vi "Autonomous Independent.vi"() -> ()   [LabVIEW 2016]
doc: "This VI is called when autonomous begins, and will automatically be terminated when autonomous ends. You can carry out timed or sensor driven robot movement independently without needing to return to the caller."
uses:
  <vilib>/Rock Robotics/WPI/Utilities/WPI_GetSetVariantRefNum.vi
  <vilib>/Rock Robotics/Network Tables/NT Write Numeric Array.vi
  Robot Global Data.vi
  <vilib>/Rock Robotics/Network Tables/NT Read String.vi
  <vilib>/Rock Robotics/WPI/RobotDrive/WPI_RobotDriveArcadeDrive_Standard(NoSaturation).vi
panel:
  out "Current Movement, for debugging":T1 {"Y Joystick Value" scale=1.0..-1.0; "X Joystick Value" scale=-1.0..1.0}
  in  "Array of robot movements":T2(array[cluster])=[{"X Joystick Value"=0.39393939393939403, "Y Joystick Value"=0.0, "Delay (sec)"=1.0, "Movement Name"="turn"}, {"X Joystick Value"=-0.3737373737373737, "Y Joystick Value"=0.0, "Delay (sec)"=1.0, "Movement Name"="turn back"}] {"Y Joystick Value" scale=1.0..-1.0; "X Joystick Value" scale=-1.0..1.0}
  # "Be sure to right-click and choose Data Operations>>Make Current Value default if you want to save the array values with the VI"
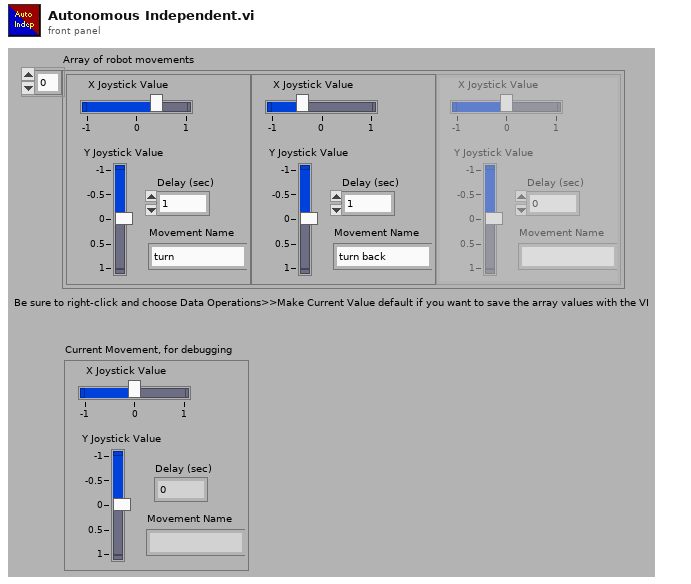
[diagram p1: front panel]
types:
  T1 = cluster{"X Joystick Value":dbl, "Y Joystick Value":dbl, "Delay (sec)":dbl, "Movement Name":string}
  T2 = cluster{"X Joystick Value":dbl, "Y Joystick Value":dbl, "Delay (sec)":dbl, "Movement Name":string}[]
  T3 = cluster{"Current Gear":enum16{"Low", "High"}, "Gear Shift State":enum16{"Low", "Shifting", "High"}}
  T4 = cluster{"Current Position":enum16{"Closed", "Open"}, "Current State":enum16{"Closed", "Shifting", "Open"}}
  T5 = typedef "WPI_RobotDriveDevRef.ctl" = cluster{"DevStatus":errorcluster, "Motors[]":T6[], "Square Inputs":bool, "Max Output":dbl}
  T6 = typedef "WPI_MotorControlDeviceRef.ctl" = cluster{"DeviceStatus":errorcluster, "Type":T7, "PWM":cluster{"PWM Channel":T8, "DeadBand":T9}, "CAN":cluster{"Device Number":u8, "SetOutput VI Ref":variant, "GetOutput VI Ref":variant, "Enable VI Ref":variant, "Disable VI Ref":variant, "Data":variant}, "Invert":bool}
  T7 = typedef "WPI_MotorControlType.ctl" = enum16{"PWM", "CAN"}
  T8 = typedef "FPGA_DIOPWMChannel.ctl" = enum8{"PWM 0", "PWM 1", "PWM 2", "PWM 3", "PWM 4", "PWM 5", "PWM 6", "PWM 7", "PWM 8", "PWM 9", "PWM MXP 0", "PWM MXP 1", "PWM MXP 2", "PWM MXP 3", "PWM MXP 4", "PWM MXP 5", "PWM MXP 6", "PWM MXP 7", "PWM MXP 8", "PWM MXP 9", "Invalid"}
  T9 = typedef "WPI_PWMDeadband.ctl" = cluster{"Name":string, "maxPositivePwm":i32, "minPositivePwm":i32, "centerPwm":i32, "maxNegativePwm":i32, "minNegativePwm":i32, "angularRange":u16}
  T10 = typedef "WPI_JoystickDevRef.ctl" = cluster{"Device":T11}
  T11 = typedef "WPI_JoystickDeviceEnum.ctl" = enum16{"USB 0", "USB 1", "USB 2", "USB 3", "USB 4", "USB 5"}
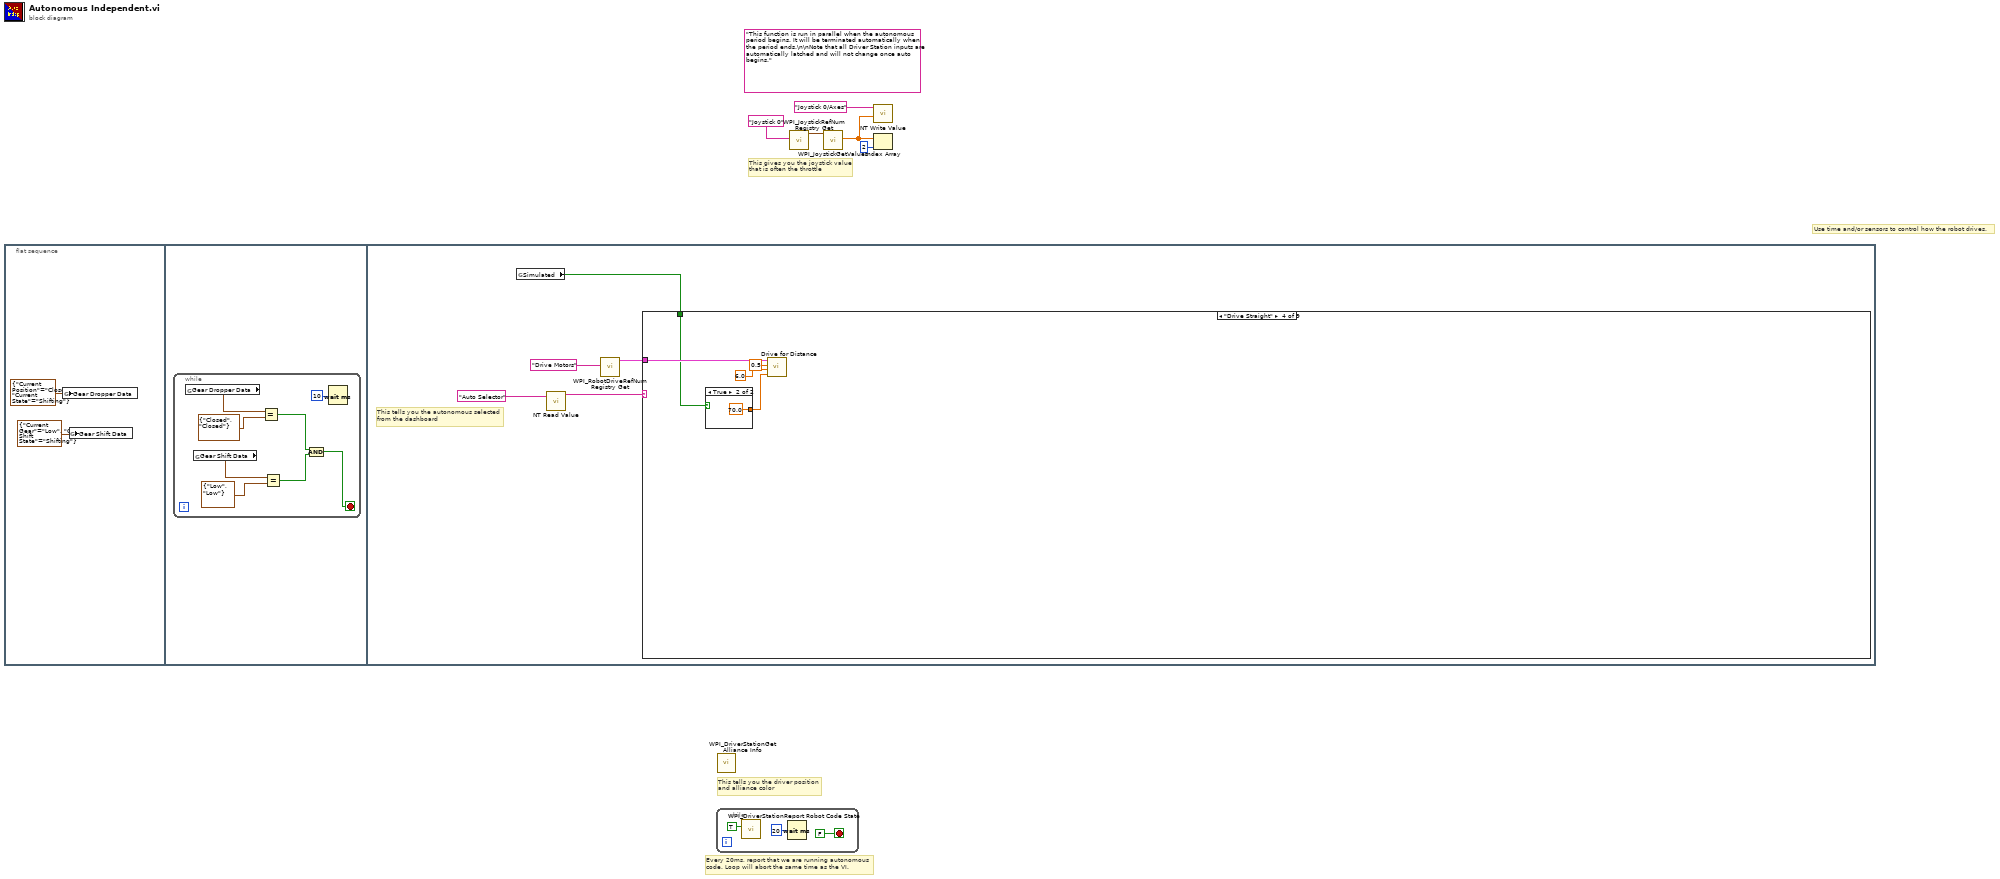
[diagram p0: block diagram]
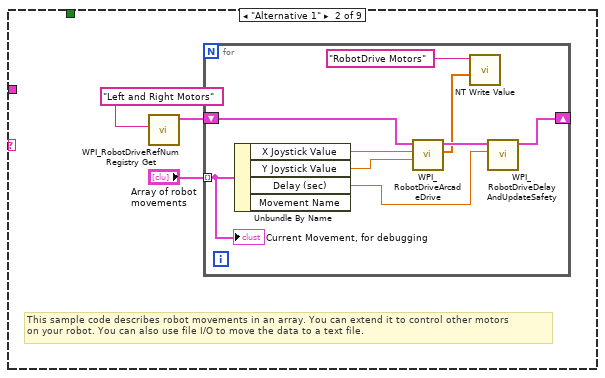
[diagram p3: hidden frame]
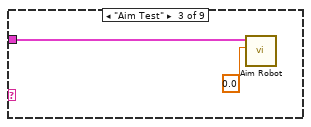
[diagram p4: hidden frame]
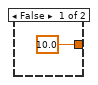
[diagram p5: hidden frame]
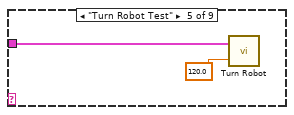
[diagram p6: hidden frame]
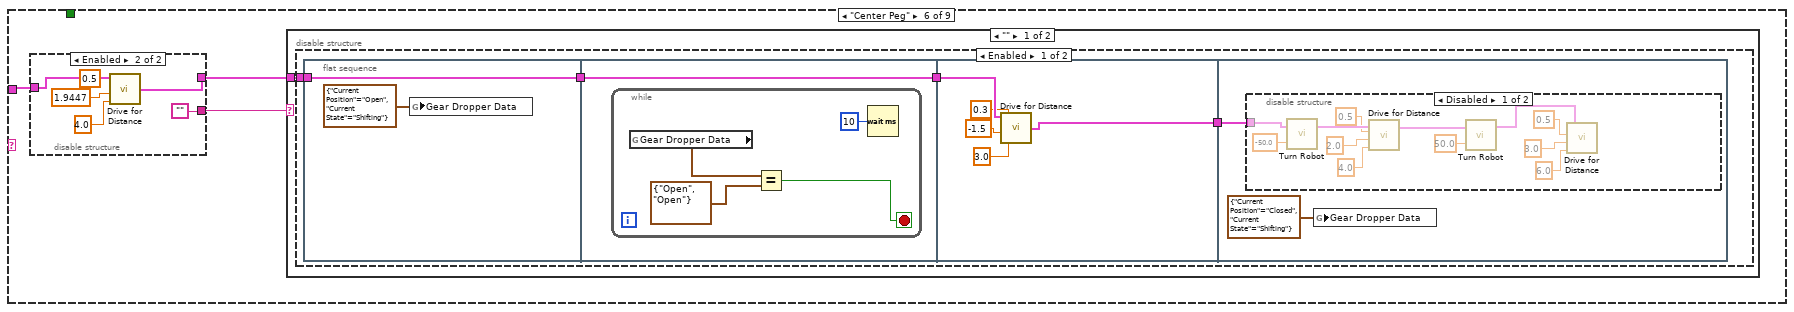
[diagram p7: hidden frame]
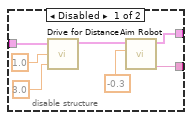
[diagram p8: hidden frame]
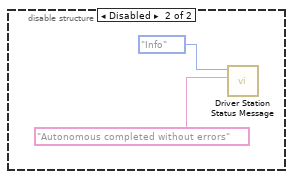
[diagram p10: hidden frame]
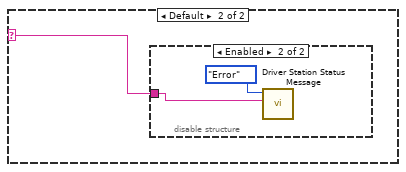
[diagram p11: hidden frame]
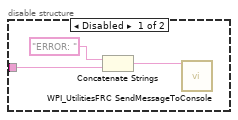
[diagram p12: hidden frame]
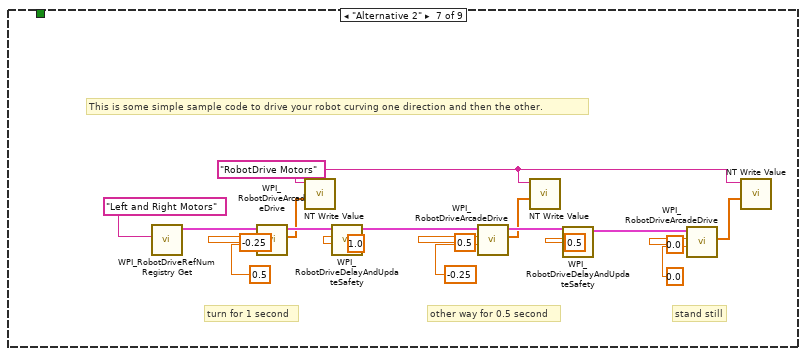
[diagram p13: hidden frame]
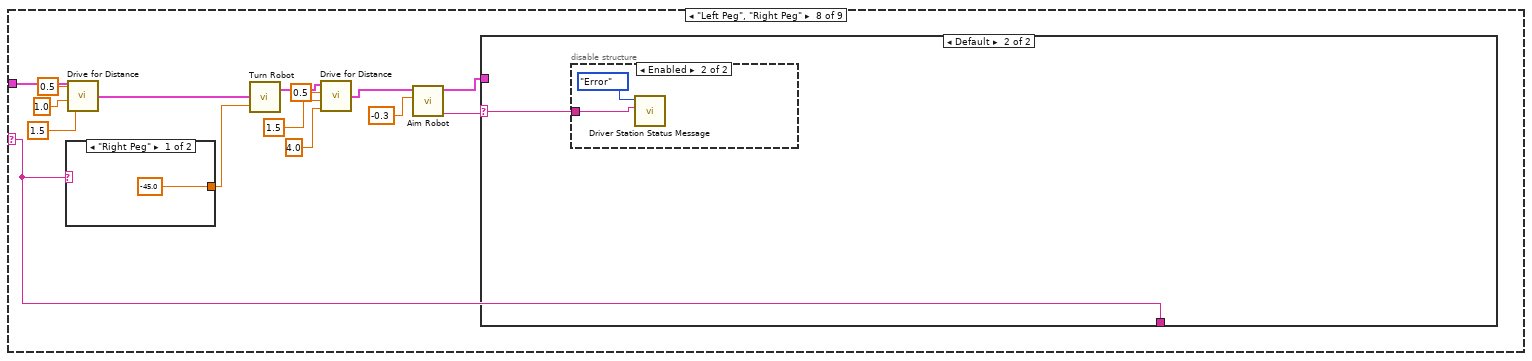
[diagram p14: hidden frame]
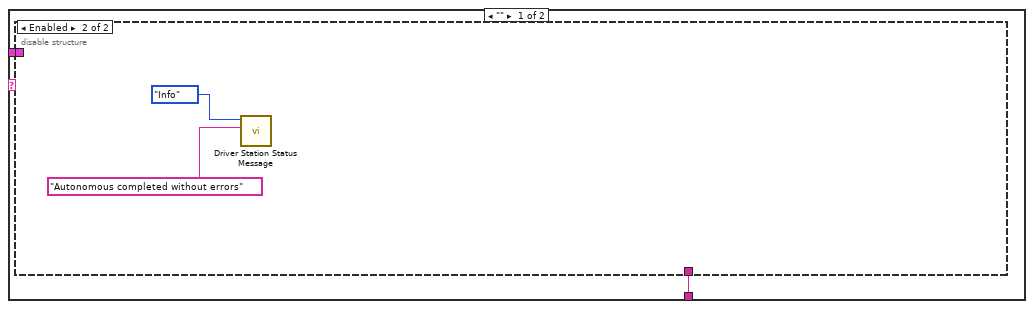
[diagram p15: hidden frame]
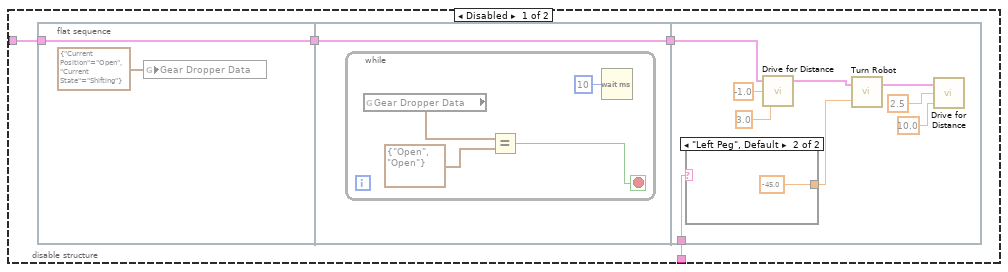
[diagram p16: hidden frame]
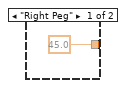
[diagram p17: hidden frame]
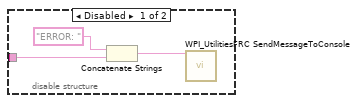
[diagram p18: hidden frame]
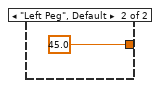
[diagram p19: hidden frame]
diagram:
  (unwired) "This function is run in parallel when the autonomous period begins. It will be terminated automatically when the period ends.\n\nNote that all Driver Station inputs are automatically latched and will not change once auto begins."
  # "Every 20ms, report that we are running autonomous\ncode. Loop will abort the same time as the VI."
  # "This gives you the joystick value\nthat is often the throttle"
  # "Use time and/or sensors to control how the robot drives."
  # "This tells you the driver position\nand alliance color"
  n1 = flat-sequence {
    frame #0 {
      n2 = global write "Robot Global Data.vi" "Gear Dropper Data"(T4 {"Current Position"=enum."Closed", "Current State"=enum."Shifting"} ("Gear Dropper Data")) -> ()
      n3 = global write "Robot Global Data.vi" "Gear Shift Data"(T3 {"Current Gear"=enum."Low", "Gear Shift State"=enum."Shifting"} ("Gear Shift Data")) -> ()
    }
    frame #1 {
      n4 = while {
        stop <- w8 stop-if-true
        n5 = global read "Robot Global Data.vi" "Gear Dropper Data"() -> (w15:T4)
        n6 = global read "Robot Global Data.vi" "Gear Shift Data"() -> (w12:T3)
        n7 = Equal?(x=w15, y=T4 {"Current Position"=enum."Closed", "Current State"=enum."Closed"}) -> (x = y?=w9:bool)
        n8 = Equal?(x=w12, y=T3 {"Current Gear"=enum."Low", "Gear Shift State"=enum."Low"}) -> (x = y?=w10:bool)
        n9 = And(x=w9, y=w10) -> (x .and. y?=w8:bool)
        n10 = Wait (ms)(milliseconds to wait=u32 10) -> ()  [unwired: 1 out]
      }
    }
    frame #2 {
      # "This tells you the autonomous selected\nfrom the dashboard"
      n11 = global read "Robot Global Data.vi" "Simulated"() -> (w16:bool)
      n12 = call-poly <vilib>:"NT Read Value.vi"("Name"="Auto Selector") -> ("String"=w18:string)  [unwired: 9 in, 1 out]
      n13 = call <vilib>:"WPI_RobotDriveRefNum Registry Get.vi"("refnum name"="Drive Motors") -> ("RobotDriveDevRef"=w20:T5)  [unwired: 9 in, 1 out]
      n14 = case shown="\"Drive Straight\"" w18 {
        selector: w18 -> [_ _ _ _ _ _ _ w124 _]
        tunnel: w20 -> [_ _ w33 w39 w43 w46 _ w129 _]
        tunnel: w16 -> [_ _ _ w35 _ _ _ _ _]
        frame Default {
          # "You can put your main auto here, or you can right-click on the case and make any\nother frame be the default case."
          # "This is the frame that will execute if no selection is made, or if it is not recognized"
        }
        frame "Alternative 1" {
          # "This sample code describes robot movements in an array. You can extend it to control other motors\non your robot. You can also use file I/O to move the data to a text file."
          n15 = call <vilib>:"WPI_RobotDriveRefNum Registry Get.vi"("refnum name"="Left and Right Motors") -> ("RobotDriveDevRef"=w22:T5)  [unwired: 1 in, 9 out]
          n16 = for {
            shift-right: [w30] -> _
            shift-left: w22 -> [w31]
            tunnel: "Array of robot movements" -> [w26] mode=indexing
            n17 = Unbundle By Name(w26) -> ("X Joystick Value"=w29:dbl, "Y Joystick Value"=w28:dbl, "Delay (sec)"=w27:dbl)  [unwired: 1 out]
            n18 = call-poly <vilib>:"WPI_RobotDriveArcadeDrive.vi"("Y axis value"=w28, "X axis value"=w29, "RobotDriveDevRef"=w31) -> ("Motor Values"=w24:dbl[], "RobotDriveDevRef"=w32:T5)  [unwired: 1 in, 6 out]
            n19 = call-poly <vilib>:"NT Write Value.vi"("Numeric Array"=w24, "Name"="RobotDrive Motors") -> ()  [unwired: 9 in, 1 out]
            n20 = call <vilib>:"WPI_RobotDriveDelayAndUpdateSafety.vi"("Delay (s)"=w27, "RobotDriveDevRef"=w32) -> ("RobotDriveDevRef 2"=w30:T5)  [unwired: 8 in, 1 out]
            "Current Movement, for debugging" <- w26
          }
        }
        frame "Aim Test" {
          n21 = call "Aim Robot.vi"("Drive Speed"=0.0, "RobotDriveDevRef"=w33) -> ()  [unwired: 8 in, 2 out]
        }
        frame "Drive Straight" {
          n22 = case shown="True" w35 {
            tunnel: [10.0 ("Timeout (s)") 70.0 ("Timeout (s)")] -> w37
            frame False {
            }
            frame True {
            }
          }
          n23 = call "Drive for Distance.vi"("Timeout (s)"=w37, "Distance (m)"=6.0, "Max Speed"=0.5, "RobotDriveDevRef"=w39) -> ()  [unwired: 1 out]
        }
        frame "Turn Robot Test" {
          n24 = call "Turn Robot.vi"("Turn Angle"=120.0, "RobotDriveDevRef"=w43) -> ()  [unwired: 1 in, 1 out]
        }
        frame "Center Peg" {
          n25 = disable-structure shown="Enabled" {
            disable-tunnel: w46 -> [w53 w56]
            disable-tunnel: [w48 w55] -> w45
            disable-tunnel: [w47 ""] -> w44
            frame Disabled {
              n26 = call "Drive for Distance.vi"("Timeout (s)"=3.0, "Distance (m)"=1.0, "RobotDriveDevRef"=w53) -> ("RobotDriveDevRef Out"=w50:T5)  [unwired: 2 in]
              n27 = call "Aim Robot.vi"("Drive Speed"=-0.3, "RobotDriveDevRef"=w50) -> ("Error Out"=w47:string, "RobotDriveDevRef Out"=w48:T5)  [unwired: 8 in]
            }
            frame Enabled {
              n28 = call "Drive for Distance.vi"("Timeout (s)"=4.0, "Distance (m)"=1.9447, "Max Speed"=0.5, "RobotDriveDevRef"=w56) -> ("RobotDriveDevRef Out"=w55:T5)
            }
          }
          n29 = case shown="\"\"" w44 {
            selector: w44 -> [_ w93]
            tunnel: w45 -> [w60 _]
            frame "" {
              n30 = disable-structure shown="Enabled" {
                disable-tunnel: w60 -> [w62 _]
                frame Enabled {
                  n31 = flat-sequence {
                    tunnel: [w65] -> w64
                    tunnel: w62 -> [w65]
                    tunnel: [w67] -> w63
                    tunnel: w64 -> [w67]
                    tunnel: w63 -> [w74]
                    tunnel: [w73] -> w61
                    tunnel: w61 -> [w77]
                    frame #0 {
                      n32 = global write "Robot Global Data.vi" "Gear Dropper Data"(T4 {"Current Position"=enum."Open", "Current State"=enum."Shifting"} ("Gear Dropper Data")) -> ()
                    }
                    frame #1 {
                      n33 = while {
                        stop <- w69 stop-if-true
                        n34 = global read "Robot Global Data.vi" "Gear Dropper Data"() -> (w71:T4)
                        n35 = Equal?(x=w71, y=T4 {"Current Position"=enum."Open", "Current State"=enum."Open"}) -> (x = y?=w69:bool)
                        n36 = Wait (ms)(milliseconds to wait=u32 10) -> ()  [unwired: 1 out]
                      }
                    }
                    frame #2 {
                      n37 = call "Drive for Distance.vi"("Timeout (s)"=3.0, "Distance (m)"=-1.5, "Max Speed"=0.3, "RobotDriveDevRef"=w74) -> ("RobotDriveDevRef Out"=w73:T5)
                    }
                    frame #3 {
                      n38 = disable-structure shown="Disabled" {
                        disable-tunnel: w77 -> [w90 _]
                        frame Disabled {
                          n39 = call "Turn Robot.vi"("Turn Angle"=-50.0, "RobotDriveDevRef"=w90) -> ("RobotDriveDevRef Out"=w88:T5)  [unwired: 1 in]
                          n40 = call "Drive for Distance.vi"("Timeout (s)"=4.0, "Distance (m)"=2.0, "Max Speed"=0.5, "RobotDriveDevRef"=w88) -> ("RobotDriveDevRef Out"=w84:T5)
                          n41 = call "Turn Robot.vi"("Turn Angle"=50.0, "RobotDriveDevRef"=w84) -> ("RobotDriveDevRef Out"=w79:T5)  [unwired: 1 in]
                          n42 = call "Drive for Distance.vi"("Timeout (s)"=6.0, "Distance (m)"=3.0, "Max Speed"=0.5, "RobotDriveDevRef"=w79) -> ()  [unwired: 1 out]
                        }
                        frame Enabled {
                        }
                      }
                      n43 = global write "Robot Global Data.vi" "Gear Dropper Data"(T4 {"Current Position"=enum."Closed", "Current State"=enum."Shifting"} ("Gear Dropper Data")) -> ()
                    }
                  }
                }
                frame Disabled {
                  n44 = call "Driver Station Status Message.vi"("Message"="Autonomous completed without errors", "Message Type"=enum16{"Error", "Warning", "Info"}."Info") -> ()  [unwired: 10 in]
                }
              }
            }
            frame Default {
              n45 = disable-structure shown="Enabled" {
                disable-tunnel: w93 -> [w94 w97]
                frame Disabled {
                  n46 = Concatenate Strings("ERROR: " ("string"), w94) -> (w95:string)
                  n47 = call <vilib>:"WPI_UtilitiesFRC SendMessageToConsole.vi"("Message"=w95) -> ()  [unwired: 14 in, 1 out]
                }
                frame Enabled {
                  n48 = call "Driver Station Status Message.vi"("Message"=w97, "Message Type"=enum16{"Error", "Warning", "Info"}."Error") -> ()  [unwired: 10 in]
                }
              }
            }
          }
        }
        frame "Alternative 2" {
          w100 = "RobotDrive Motors" ("Name")
          # "This is some simple sample code to drive your robot curving one direction and then the other."
          # "stand still"
          # "other way for 0.5 second"
          # "turn for 1 second"
          n49 = call <vilib>:"WPI_RobotDriveRefNum Registry Get.vi"("refnum name"="Left and Right Motors") -> ("RobotDriveDevRef"=w116:T5)  [unwired: 1 in, 9 out]
          n50 = call-poly <vilib>:"WPI_RobotDriveArcadeDrive.vi"("Y axis value"=0.5 ("X axis value"), "X axis value"=-0.25, "RobotDriveDevRef"=w116) -> ("Motor Values"=w99:dbl[], "RobotDriveDevRef"=w109:T5)  [unwired: 1 in, 6 out]
          n51 = call-poly <vilib>:"NT Write Value.vi"("Numeric Array"=w99, "Name"=w100) -> ()  [unwired: 9 in, 1 out]
          n52 = call <vilib>:"WPI_RobotDriveDelayAndUpdateSafety.vi"("Delay (s)"=1.0, "RobotDriveDevRef"=w109) -> ("RobotDriveDevRef 2"=w110:T5)  [unwired: 8 in, 1 out]
          n53 = call-poly <vilib>:"WPI_RobotDriveArcadeDrive.vi"("Y axis value"=-0.25 ("X axis value"), "X axis value"=0.5, "RobotDriveDevRef"=w110) -> ("Motor Values"=w101:dbl[], "RobotDriveDevRef"=w111:T5)  [unwired: 1 in, 6 out]
          n54 = call-poly <vilib>:"NT Write Value.vi"("Numeric Array"=w101, "Name"=w100) -> ()  [unwired: 9 in, 1 out]
          n55 = call <vilib>:"WPI_RobotDriveDelayAndUpdateSafety.vi"("Delay (s)"=0.5, "RobotDriveDevRef"=w111) -> ("RobotDriveDevRef 2"=w112:T5)  [unwired: 8 in, 1 out]
          n56 = call-poly <vilib>:"WPI_RobotDriveArcadeDrive.vi"("Y axis value"=0.0 ("X axis value"), "X axis value"=0.0, "RobotDriveDevRef"=w112) -> ("Motor Values"=w102:dbl[])  [unwired: 1 in, 7 out]
          n57 = call-poly <vilib>:"NT Write Value.vi"("Numeric Array"=w102, "Name"=w100) -> ()  [unwired: 9 in, 1 out]
        }
        frame "Left Peg", "Right Peg" {
          n58 = case shown="\"Right Peg\"" w124 {
            tunnel: [-45.0 45.0] -> w127
            frame "Right Peg" {
            }
            frame "Left Peg", Default {
            }
          }
          n59 = call "Drive for Distance.vi"("Timeout (s)"=1.5, "Distance (m)"=1.0, "Max Speed"=0.5, "RobotDriveDevRef"=w129) -> ("RobotDriveDevRef Out"=w128:T5)
          n60 = call "Turn Robot.vi"("Turn Angle"=w127, "RobotDriveDevRef"=w128) -> ("RobotDriveDevRef Out"=w122:T5)  [unwired: 1 in]
          n61 = call "Drive for Distance.vi"("Timeout (s)"=4.0, "Distance (m)"=1.5, "Max Speed"=0.5, "RobotDriveDevRef"=w122) -> ("RobotDriveDevRef Out"=w121:T5)
          n62 = call "Aim Robot.vi"("Drive Speed"=-0.3, "RobotDriveDevRef"=w121) -> ("Error Out"=w123:string, "RobotDriveDevRef Out"=w125:T5)  [unwired: 8 in]
          n63 = case shown="Default" w123 {
            selector: w123 -> [_ w158]
            tunnel: w125 -> [w133 _]
            tunnel: w124 -> [w132 _]
            frame "" {
              n64 = disable-structure shown="Enabled" {
                disable-tunnel: w133 -> [w135 _]
                disable-tunnel: w132 -> [w134 _]
                frame Disabled {
                  n65 = flat-sequence {
                    tunnel: [w138] -> w137
                    tunnel: w135 -> [w138]
                    tunnel: [w140] -> w136
                    tunnel: w137 -> [w140]
                    tunnel: w136 -> [w147]
                    tunnel: w134 -> [w145]
                    frame #0 {
                      n66 = global write "Robot Global Data.vi" "Gear Dropper Data"(T4 {"Current Position"=enum."Open", "Current State"=enum."Shifting"} ("Gear Dropper Data")) -> ()
                    }
                    frame #1 {
                      n67 = while {
                        stop <- w142 stop-if-true
                        n68 = global read "Robot Global Data.vi" "Gear Dropper Data"() -> (w144:T4)
                        n69 = Equal?(x=w144, y=T4 {"Current Position"=enum."Open", "Current State"=enum."Open"}) -> (x = y?=w142:bool)
                        n70 = Wait (ms)(milliseconds to wait=u32 10) -> ()  [unwired: 1 out]
                      }
                    }
                    frame #2 {
                      n71 = case shown="\"Left Peg\", Default" w145 {
                        tunnel: [45.0 -45.0] -> w146
                        frame "Right Peg" {
                        }
                        frame "Left Peg", Default {
                        }
                      }
                      n72 = call "Drive for Distance.vi"("Timeout (s)"=3.0, "Distance (m)"=-1.0, "RobotDriveDevRef"=w147) -> ("RobotDriveDevRef Out"=w151:T5)  [unwired: 2 in]
                      n73 = call "Turn Robot.vi"("Turn Angle"=w146, "RobotDriveDevRef"=w151) -> ("RobotDriveDevRef Out"=w150:T5)  [unwired: 1 in]
                      n74 = call "Drive for Distance.vi"("Timeout (s)"=10.0, "Distance (m)"=2.5, "RobotDriveDevRef"=w150) -> ()  [unwired: 2 in, 1 out]
                    }
                  }
                }
                frame Enabled {
                  n75 = call "Driver Station Status Message.vi"("Message"="Autonomous completed without errors", "Message Type"=enum16{"Error", "Warning", "Info"}."Info") -> ()  [unwired: 10 in]
                }
              }
            }
            frame Default {
              n76 = disable-structure shown="Enabled" {
                disable-tunnel: w158 -> [w159 w163]
                frame Disabled {
                  n77 = Concatenate Strings("ERROR: " ("string"), w159) -> (w160:string)
                  n78 = call <vilib>:"WPI_UtilitiesFRC SendMessageToConsole.vi"("Message"=w160) -> ()  [unwired: 14 in, 1 out]
                }
                frame Enabled {
                  n79 = call "Driver Station Status Message.vi"("Message"=w163, "Message Type"=enum16{"Error", "Warning", "Info"}."Error") -> ()  [unwired: 10 in]
                }
              }
            }
          }
        }
        frame "Your Turn" {
        }
      }
    }
  }
  n80 = while {
    stop <- FALSE stop-if-true
    n81 = call <vilib>:"WPI_DriverStationReport Robot Code State.vi"("Autonomous"=TRUE) -> ()  [unwired: 10 in, 1 out]
    n82 = Wait (ms)(milliseconds to wait=u32 20) -> ()  [unwired: 1 out]
  }
  n83 = call <vilib>:"WPI_DriverStationGet Alliance Info.vi"() -> ()  [unwired: 12 out]
  n84 = call <vilib>:"WPI_JoystickRefNum Registry Get.vi"("refnum name"="Joystick 0") -> ("JoystickDevRef"=w4:T10)  [unwired: 1 in, 9 out]
  n85 = call <vilib>:"WPI_JoystickGetValues.vi"("JoystickDevRef"=w4) -> ("Axes"=w2:dbl[])  [unwired: 6 in, 4 out]
  n86 = call-poly <vilib>:"NT Write Value.vi"("Numeric Array"=w2, "Name"="Joystick 0/Axes") -> ()  [unwired: 9 in, 1 out]
  n87 = Index Array(array=w2, index=2) -> ()  [unwired: 1 out]
